vi "Drag Ended.vi"(8 "error in (no error)":errorcluster, 11 "BetterTreeHandle in":refnum<class "BetterTreeHandle.lvclass">) -> (0 "error out":errorcluster, 3 "BetterTreeHandle out":refnum<class "BetterTreeHandle.lvclass">)   [LabVIEW 2020, in "BetterDragAndDrop.lvlib" / "BetterTreeHandle.lvclass"]
uses:
  BetterTreeHandle.lvclass
  BetterTreeHandle.lvclass/BetterTreeHandle.ctl
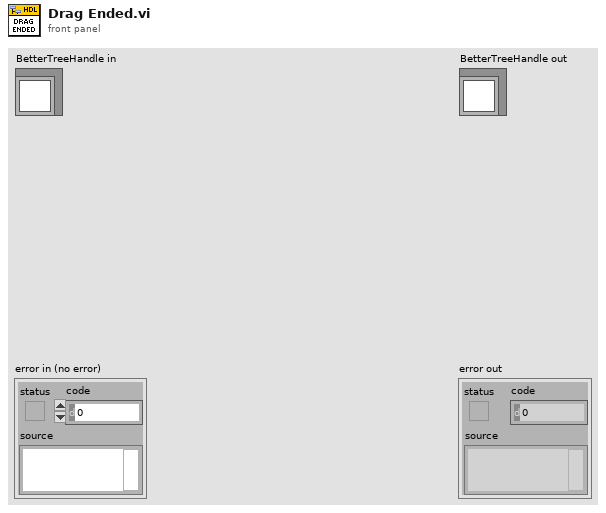
[diagram p1: front panel]
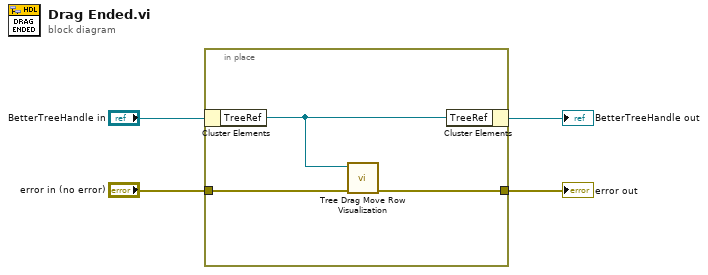
[diagram p0: block diagram]
diagram:
  n1 = in-place {
    in-place-border: "error in (no error)" -> [w7]
    in-place-border: [w6] -> w2
    n2 = in-place-cluster #1("BetterTreeHandle in") -> ("TreeRef"=w5:refnum<vi>)
    n3 = call "Tree Drag Move Row Visualization.vi"("error in (no error)"=w7, "TreeRef"=w5) -> ("error out"=w6:errorcluster)  [unwired: 9 in]
    n4 = in-place-cluster #1("TreeRef"=w5) -> (→"BetterTreeHandle out":refnum<class "BetterTreeHandle.lvclass">)
  }
  "error out" <- w2
